vi "Get Installed Software extended.vi"(8 "error in (no error)":errorcluster, 9 "Cached (F)":bool, 10 "Item Types (all visible)":T3 items=["all visible", "all including hidden", "standard only", "startup only"], 11 "Session in":refnum<k21>) -> (0 "error out":errorcluster, 2 "Software Components":T1[](array[typedef]) {"Visibility Type" items=["standard", "hidden", "system", "unknown", "startup", "image"]}, 3 "Session out":refnum<k21>)   [LabVIEW 2014, in "nisyscfg.lvlib"]
uses:
  nisyscfg.lvlib
  Component Types.ctl
  Software Extended.ctl
  Component Type.ctl
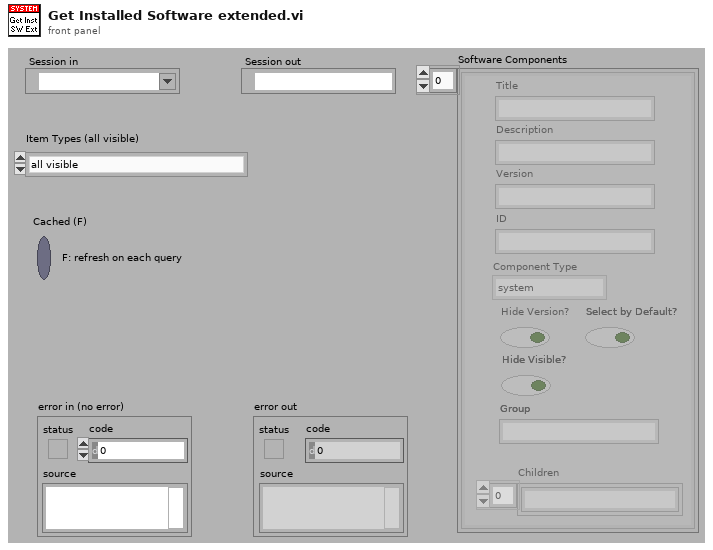
[diagram p1: front panel]
types:
  T1 = typedef "nisyscfg.lvlib/Software Extended.ctl" = cluster{"Description":string, "ID":string, "Version":string, "Title":string, "Visibility Type":T2, "Hide Version?":bool, "Children":string[], "Select by Default?":bool, "Hide Visible?":bool, "Group":string}
  T2 = typedef "nisyscfg.lvlib/Component Type.ctl" = u32
  T3 = typedef "nisyscfg.lvlib/Component Types.ctl" = u32
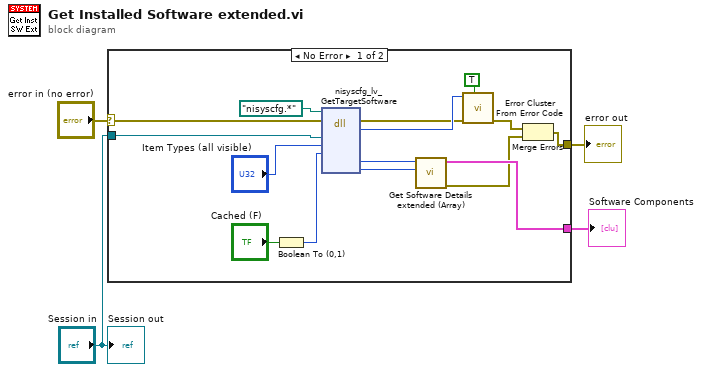
[diagram p0: block diagram]
diagram:
  n1 = case shown="No Error" "error in (no error)" {
    selector: "error in (no error)" -> [w16 w20]
    tunnel: [w8 w20] -> w4
    tunnel: "Session in" -> [w15 _]
    tunnel: [w11 _] -> w2
    frame No Error {
      n2 = Boolean To (0,1)(Boolean="Cached (F)") -> (0, 1=w17:i16)
      n3 = dll-call lib="nisyscfg.*" fn="nisyscfg_lv_GetTargetSoftware" label="GetTargetSoftware"(path in=path "nisyscfg.*", error in=w16, "system"=w15, "includeTypes"="Item Types (all visible)", "cached"=w17) -> (error out=w7:errorcluster, "result"=w19:i32, "softwareEnum"=w12:u64, "numComponents"=w10:i32)  [unwired: 6 in, 1 out]
      n4 = call "Get Software Details extended (Array).vi"("Number of Elements"=w10, "Enumerator in"=w12) -> ("error out"=w5:errorcluster, "Software Components"=w11:T1[])  [unwired: 8 in]
      n5 = call "Error Cluster From Error Code.vi"("show call chain? (False)"=TRUE, "error in (no error)"=w7, "error code (0)"=w19) -> ("error out"=w6:errorcluster)  [unwired: 6 in]
      n6 = Merge Errors(w6, w5) -> (w8:errorcluster)
    }
    frame Error {
    }
  }
  "error out" <- w4
  "Software Components" <- w2
  "Session out" <- "Session in"
